vi "Pneumatic Blink Deflicker Test.vi"() -> ()   [LabVIEW 2013]
uses:
  Robot Code/Utilities/TimeManager.vi
  Common Code/Change Detect.vi
  Common Code/Change Detect Boolean.vi
panel:
  in  "Limit to Blink":bool
  in  "stop":bool
  out "Filtered Output":bool
  in  "Deflicker":dbl format="%#_13g"
  in  "Blink":dbl format="%#_13g"
  in  "In":bool
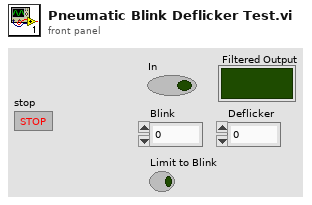
[diagram p1: front panel]
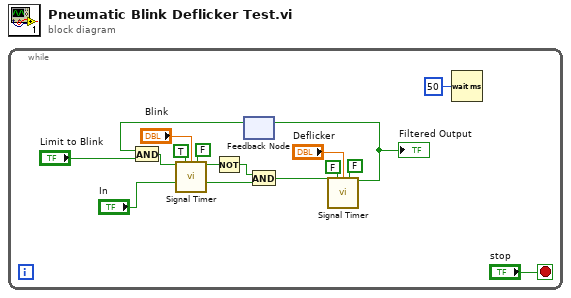
[diagram p0: block diagram]
diagram:
  n1 = while {
    stop <- "stop" stop-if-true
    n2 = feedback #1() -> (w7:bool)  [unwired: 1 in]
    n3 = And(x=w7, y="Limit to Blink") -> (x .and. y?=w8:bool)
    n4 = call "Signal Timer.vi"("Input"=w8, "Edge"=TRUE, "Interval"="Blink", "Pull"=FALSE ("Edge")) -> ("Filtered Output"=w12:bool)  [unwired: 11 in]
    n5 = Not(x=w12) -> (.not. x?=w11:bool)
    n6 = And(x=w11, y="In") -> (x .and. y?=w9:bool)
    n7 = call "Signal Timer.vi"("Input"=w9, "Edge"=FALSE, "Interval"="Deflicker", "Pull"=FALSE ("Edge")) -> ("Filtered Output"=w10:bool)  [unwired: 11 in]
    "Filtered Output" <- w10
    n8 = feedback-in #1(w10) -> ()
    n9 = Wait (ms)(milliseconds to wait=u32 50) -> ()  [unwired: 1 out]
  }
